vi "Building_Subtrack_Add_Part_till_Normal_Point-1.vi"(4 "[IN] Last Normal Poi\nnt after 101 Problem":i32, 5 "[IN] # Track with \n101 Problem Point":i32, 6 "[IN] Index of \nPoint after 101":i32, 7 "error IN":errorcluster, 8 "[IN] Subtrack":T1, 9 "[IN] Last Point in Subtrack":i32, 10 "[IN] Still connected\ntracks in group":T2) -> (0 "error OUT":errorcluster, 1 "[OUT] Subtrack":T1, 2 "[OUT] Last point in subtrack":i32)   [LabVIEW 2013]
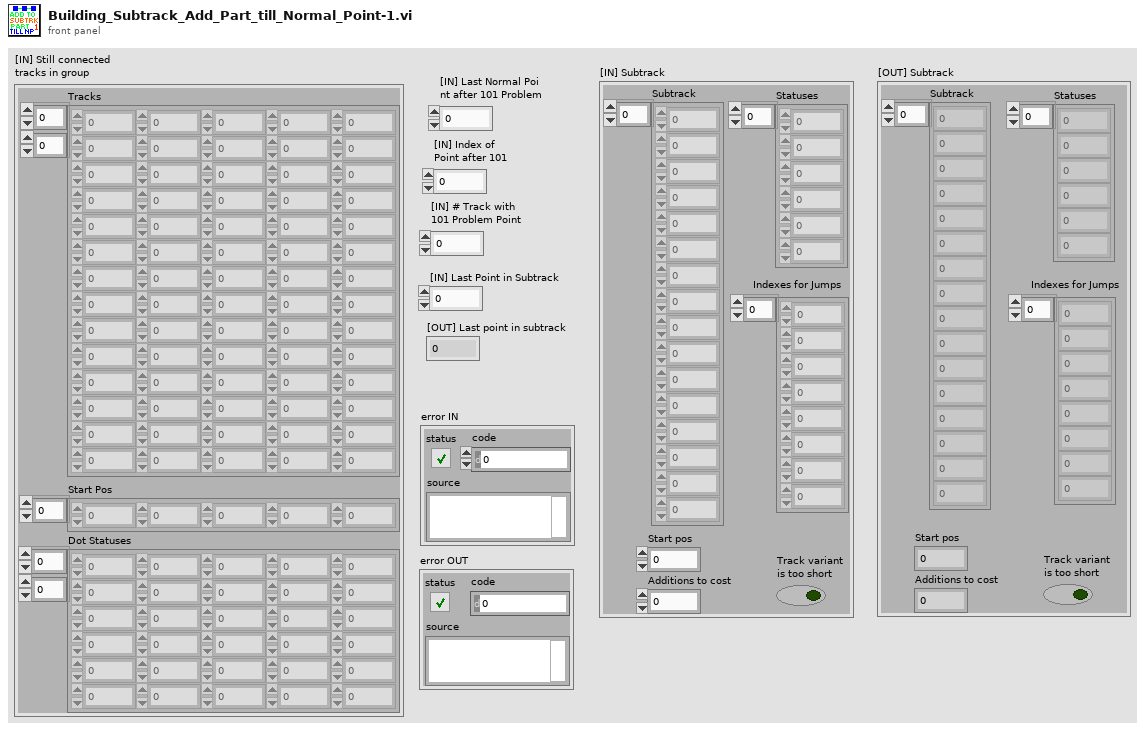
[diagram p1: front panel]
types:
  T1 = cluster{"Subtrack":dbl[], "Statuses":i16[], "Start pos":i32, "Additions to cost":i8, "Track variant \nis too short":bool, "Indexes for Jumps":i32[]}
  T2 = cluster{"Tracks":dbl[][], "Start Pos":i32[], "Dot Statuses":i16[][]}
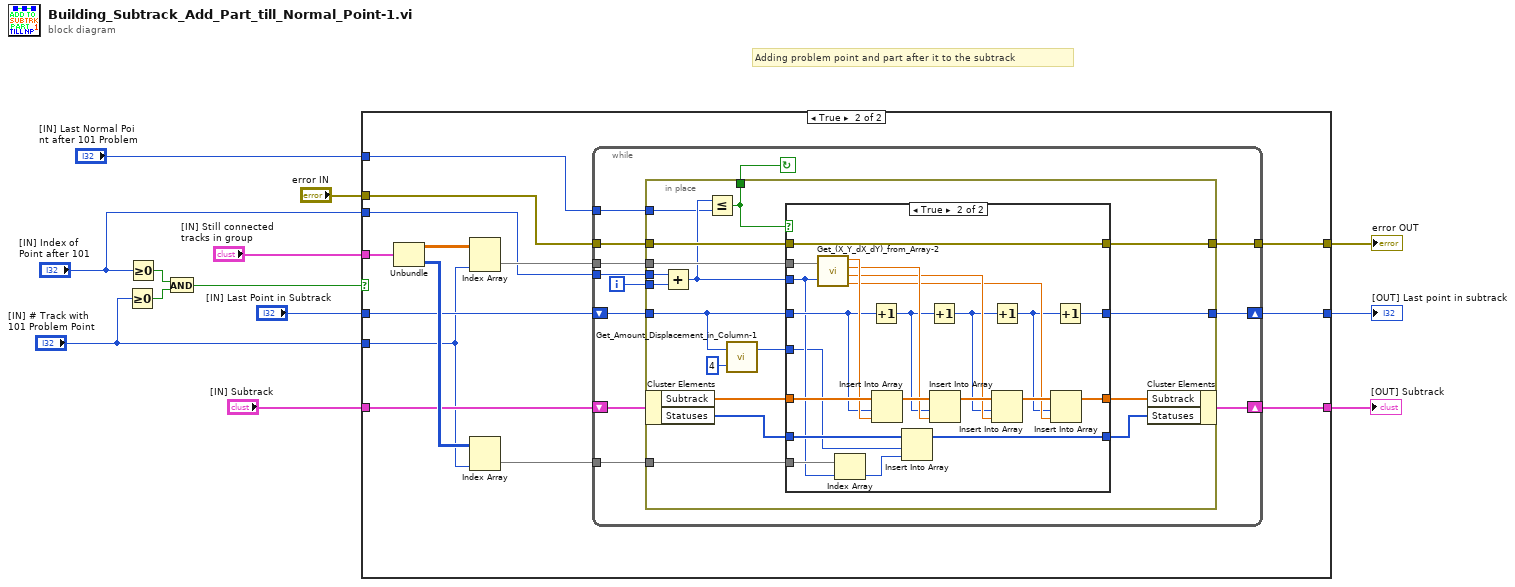
[diagram p0: block diagram]
diagram:
  # "Adding problem point and part after it to the subtrack"
  n1 = Greater Or Equal To 0?(x="[IN] # Track with \n101 Problem Point") -> (x >= 0?=w7:bool)
  n2 = Greater Or Equal To 0?(x="[IN] Index of \nPoint after 101") -> (x >= 0?=w8:bool)
  n3 = And(x=w8, y=w7) -> (x .and. y?=w6:bool)
  n4 = case shown="True" w6 {
    tunnel: "[IN] Still connected\ntracks in group" -> [_ w30]
    tunnel: [w14 w26] -> w12
    tunnel: [w16 w25] -> w11
    tunnel: "[IN] Subtrack" -> [w15 w24]
    tunnel: [w15 w23] -> w9
    tunnel: "[IN] # Track with \n101 Problem Point" -> [_ w19]
    tunnel: "error IN" -> [w16 w22]
    tunnel: "[IN] Last Point in Subtrack" -> [w14 w21]
    tunnel: "[IN] Index of \nPoint after 101" -> [_ w18]
    tunnel: "[IN] Last Normal Poi\nnt after 101 Problem" -> [_ w17]
    frame False {
    }
    frame True {
      n5 = Unbundle(w30) -> ("Tracks"=w29:dbl[][], "Dot Statuses"=w27:i16[][])  [unwired: 1 out]
      n6 = Index Array(array=w29, index (col)=w19) -> (element=w28:dbl[])  [unwired: 1 in]
      n7 = Index Array(array=w27, index (col)=w19) -> (element=w20:i16[])  [unwired: 1 in]
      n8 = while {
        tunnel: w28 -> [w42]
        tunnel: w20 -> [w40]
        shift-right: [w33] -> w23
        shift-left: w24 -> [w34]
        tunnel: w22 -> [w38]
        tunnel: [w37] -> w25
        shift-right: [w36] -> w26
        shift-left: w21 -> [w35]
        tunnel: w18 -> [w32]
        tunnel: w17 -> [w31]
        i -> [w39]
        stop <- w41 continue-if-true
        n9 = in-place {
          in-place-border: w42 -> [w59]
          in-place-border: [w58] -> w41
          in-place-border: w40 -> [w57]
          in-place-border: w39 -> [w45]
          in-place-border: w38 -> [w56]
          in-place-border: [w55] -> w37
          in-place-border: [w54] -> w36
          in-place-border: w35 -> [w52]
          in-place-border: w32 -> [w46]
          in-place-border: w31 -> [w43]
          n10 = in-place-cluster #1(w34) -> ("Subtrack"=w50:dbl[], "Statuses"=w49:i16[])
          n11 = Add(x=w46, y=w45) -> (x+y=w44:i32)
          n12 = Less Or Equal?(x=w44, y=w43) -> (x <= y?=w58:bool)
          n13 = call "Get_Amount_Displacement_in_Column-1.vi"("multiplier"=4, "# Rows"=w52) -> ("Displ amount"=w51:i32)  [unwired: 1 out]
          n14 = case shown="True" w58 {
            tunnel: w59 -> [_ w85]
            tunnel: w50 -> [w62 w84]
            tunnel: w52 -> [w60 w82]
            tunnel: w44 -> [_ w71]
            tunnel: w49 -> [w63 w73]
            tunnel: w57 -> [_ w72]
            tunnel: [w62 w69] -> w48
            tunnel: [w63 w68] -> w47
            tunnel: w56 -> [w61 w67]
            tunnel: [w61 w67] -> w55
            tunnel: [w60 w64] -> w54
            tunnel: w51 -> [_ w66]
            frame False {
            }
            frame True {
              n15 = call "Get_(X_Y_dX_dY)_from_Array-2.vi"("(X,Y,dX,dY)"=w85, "Index of Displacement"=w71) -> ("X"=w83:dbl, "Y"=w80:dbl, "dX"=w77:dbl, "dY"=w74:dbl)
              n16 = Index Array(array=w72, index=w71) -> (element=w70:i16)
              n17 = Increment(x=w82) -> (x+1=w78:i32)
              n18 = Insert Into Array(array=w84, index=w82, new element=w83) -> (w81:dbl[])
              n19 = Insert Into Array(array=w73, index=w66, new element=w70) -> (w68:i16[])
              n20 = Increment(x=w78) -> (x+1=w76:i32)
              n21 = Insert Into Array(array=w81, index=w78, new element=w80) -> (w79:dbl[])
              n22 = Increment(x=w76) -> (x+1=w65:i32)
              n23 = Insert Into Array(array=w79, index=w76, new element=w77) -> (w75:dbl[])
              n24 = Insert Into Array(array=w75, index=w65, new element=w74) -> (w69:dbl[])
              n25 = Increment(x=w65) -> (x+1=w64:i32)
            }
          }
          n26 = in-place-cluster #1("Subtrack"=w48, "Statuses"=w47) -> (w33:T1)
        }
      }
    }
  }
  "[OUT] Last point in subtrack" <- w12
  "error OUT" <- w11
  "[OUT] Subtrack" <- w9
